vi "Decimate and Interpolate (multiple).vi"(8 "error in (no error)":errorcluster, 11 "Multiple XY-data in":cluster{"X-array":dbl[], "Y-array":dbl[]}[](array[cluster]) {"Y-array" format="%.2p"; "X-array" format="%.2p"}) -> (0 "error out":errorcluster, 3 "Multiple XY-data out":cluster{"X-array":dbl[], "Y-array":dbl[]}[](array[cluster]) {"Y-array" format="%.2p"; "X-array" format="%.2p"})   [LabVIEW 2016, in "xy_utilities.lvlib"]
uses:
  xy_utilities.lvlib
panel:
  in  "Configure":T1={"X Low"=0.05, "X High"=0.5, "X Step"=0.01, "fake point value"=0.05} {"fake point value" format="%#_6p"; "X Step" format="%#_6p"; "X High" format="%#_6p"; "X Low" format="%#_6p"}
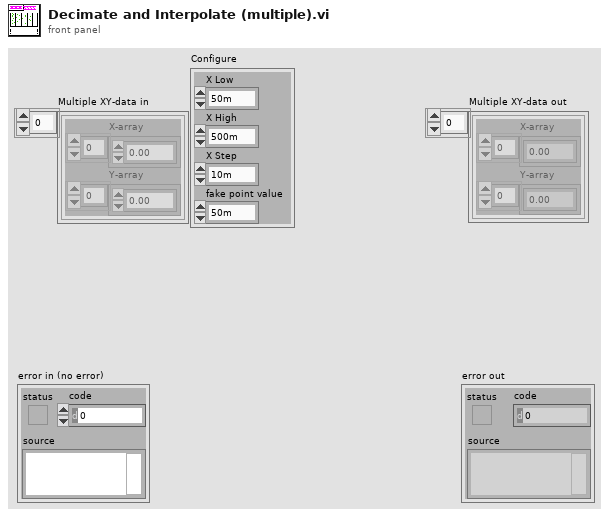
[diagram p1: front panel]
types:
  T1 = cluster{"X Low":dbl, "X High":dbl, "X Step":dbl, "fake point value":dbl}
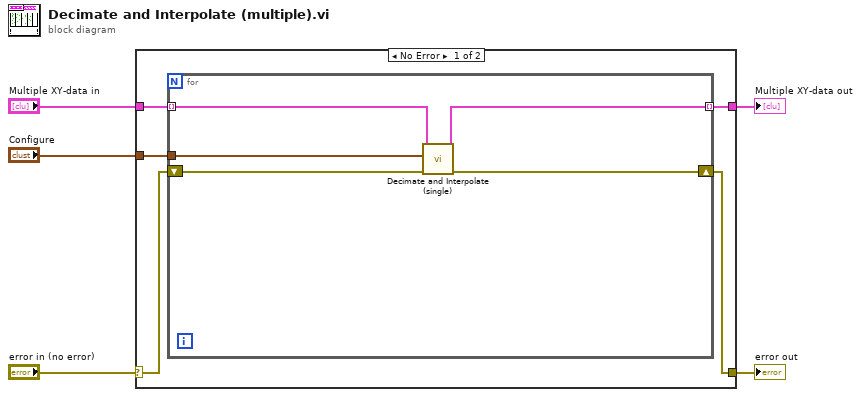
[diagram p0: block diagram]
diagram:
  n1 = case shown="No Error" "error in (no error)" {
    selector: "error in (no error)" -> [w8 w17]
    tunnel: [w7 w17] -> w4
    tunnel: "Multiple XY-data in" -> [w10 w16]
    tunnel: [w9 w16] -> w2
    tunnel: "Configure" -> [w6 _]
    frame No Error {
      n2 = for {
        tunnel: w10 -> [w15] mode=indexing
        tunnel: [w12] -> w9 mode=indexing
        shift-right: [w13] -> w7
        shift-left: w8 -> [w14]
        tunnel: w6 -> [w11]
        n3 = call "Decimate and Interpolate (single).vi"("error in (no error)"=w14, "Configure"=w11, "XY-data in"=w15) -> ("error out"=w13:errorcluster, "XY-data out"=w12:cluster{"X-array":dbl[], "Y-array":dbl[]})  [unwired: 7 in]
      }
    }
    frame Error {
    }
  }
  "error out" <- w4
  "Multiple XY-data out" <- w2
